vi "PS_set_field_rate.vi"(0 "ramping rate":variant, 1 "set point":variant, 2 "Power supply":T1(ring)) -> ()   [LabVIEW 2020]
panel:
  out "error IO":errorcluster
  in  "error in (no error)":errorcluster
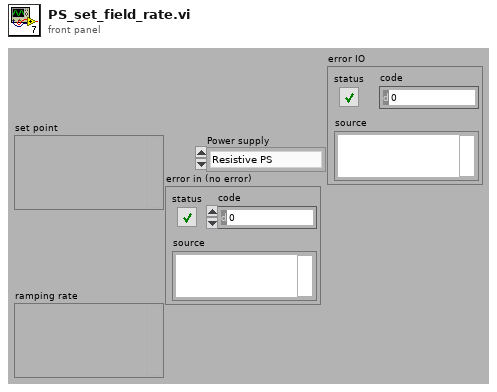
[diagram p1: front panel]
types:
  T1 = enum16{"Resistive PS", "SCM2 PS", "SCM1 PS", "Generic PS", "PPMS"}
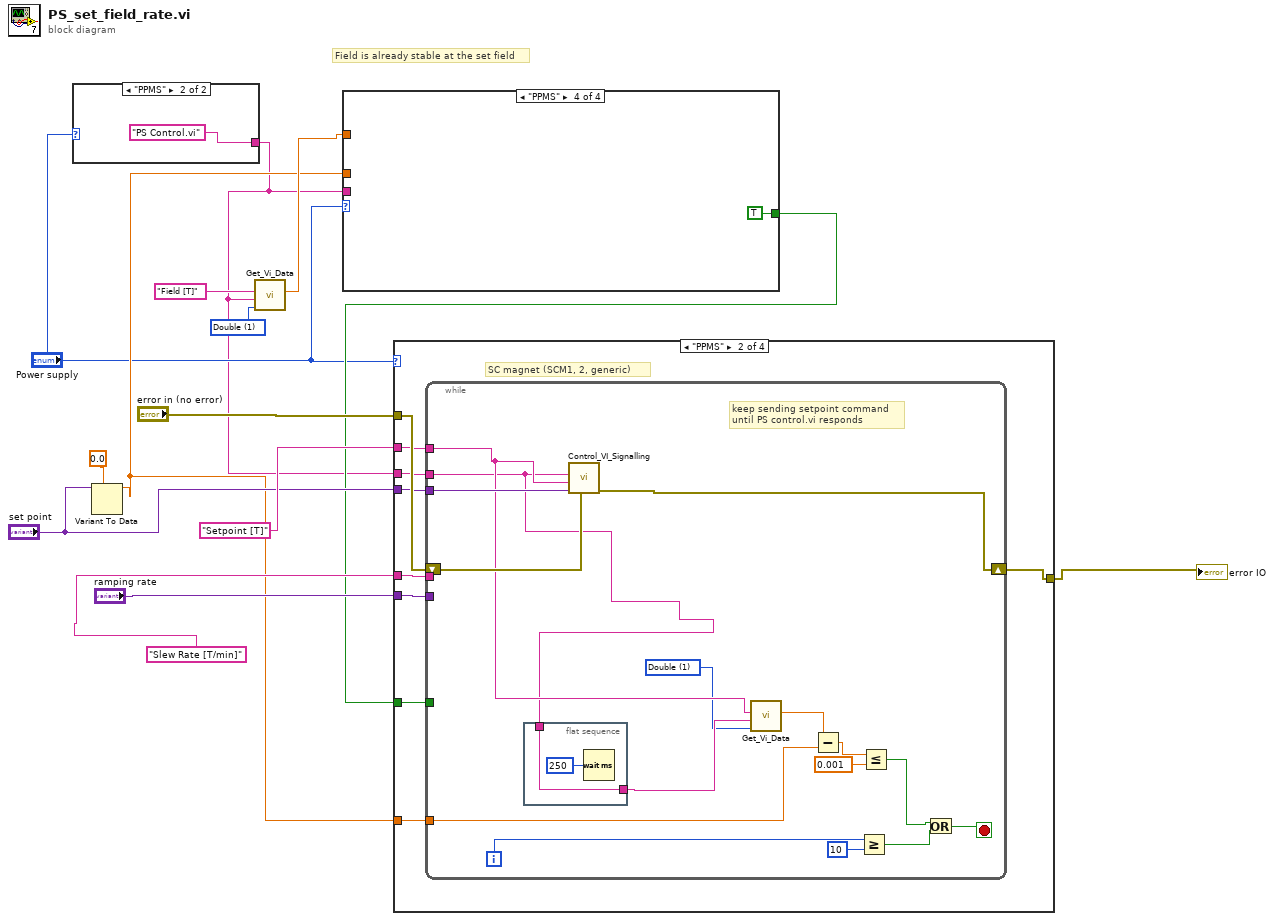
[diagram p0: block diagram]
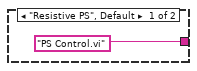
[diagram p2: hidden frame]
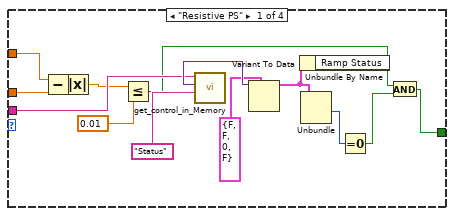
[diagram p3: hidden frame]
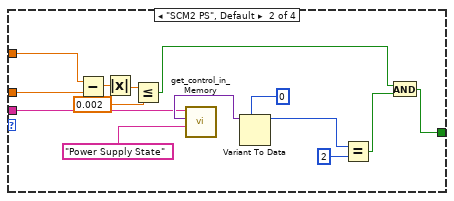
[diagram p4: hidden frame]
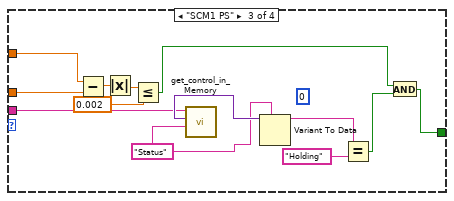
[diagram p5: hidden frame]
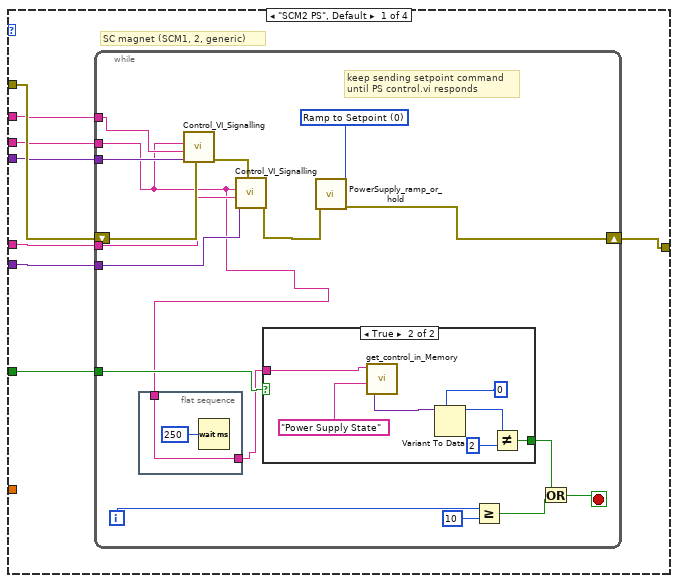
[diagram p6: hidden frame]
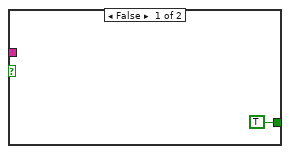
[diagram p7: hidden frame]
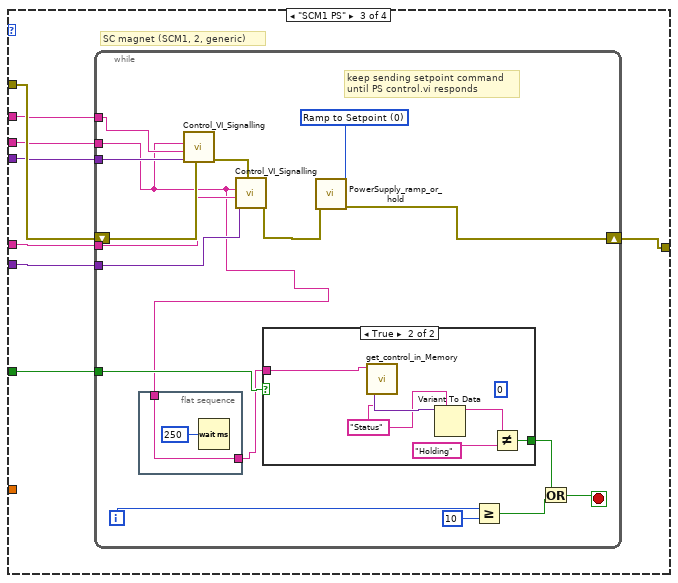
[diagram p8: hidden frame]
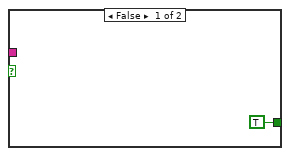
[diagram p9: hidden frame]
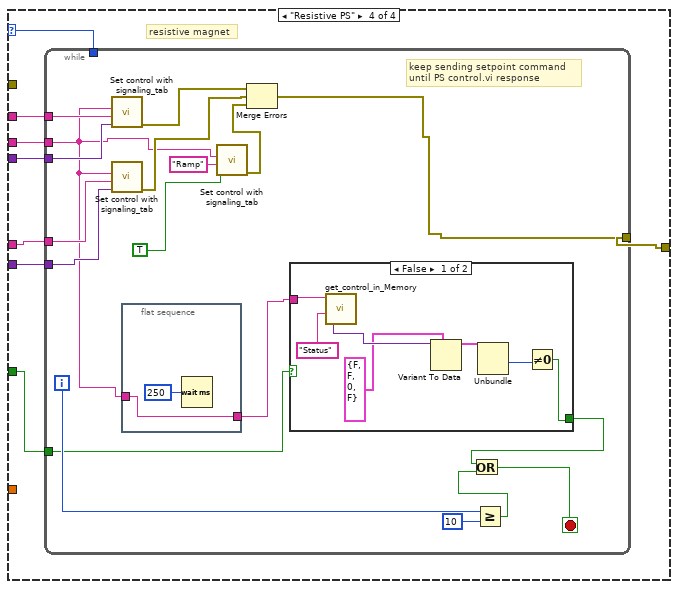
[diagram p10: hidden frame]
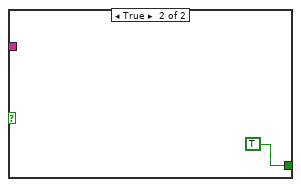
[diagram p11: hidden frame]
diagram:
  w10 = u16 1 items=["String", "Double", "Boolean", "Variant"] ("Data Type")
  # "Field is already stable at the set field"
  n1 = case shown="\"PPMS\"" "Power supply" {
    tunnel: ["PS Control.vi" ("VI name") "PS Control.vi" ("VI name")] -> w1
    frame "Resistive PS", Default {
    }
    frame "PPMS" {
    }
  }
  n2 = Variant To Data(type=0.0, Variant="set point") -> (data=w3:dbl)  [unwired: 1 in, 1 out]
  n3 = call "Get_Vi_Data.vi"("Data Type"=w10, "VI name"=w1, "Control Name"="Field [T]") -> ("Data (Double)"=w6:dbl)  [unwired: 4 in, 4 out]
  n4 = case shown="\"PPMS\"" "Power supply" {
    tunnel: w1 -> [w28 w41 w56 _]
    tunnel: [w27 w37 w54 TRUE] -> w5
    tunnel: w6 -> [w26 w36 w53 _]
    tunnel: w3 -> [w25 w35 w52 _]
    frame "Resistive PS" {
      n5 = Subtract(x=w26, y=w25) -> (x-y=w24:dbl)
      n6 = Absolute Value(x=w24) -> (abs(x)=w20:dbl)
      n7 = Less Or Equal?(x=w20, y=0.01) -> (x <= y?=w22:bool)
      n8 = call "get_control_in_Memory.vi"("Control Name"="Status", "VI Name"=w28) -> ("Value"=w29:variant)  [unwired: 2 in, 1 out]
      n9 = Variant To Data(type=cluster{bool, bool, "Ramp Status":u16, bool} {FALSE, FALSE, "Ramp Status"=0, FALSE} ("Status"), Variant=w29) -> (data=w19:cluster{bool, bool, "Ramp Status":u16, bool})  [unwired: 1 in, 1 out]
      n10 = Unbundle By Name(w19) -> ()  [unwired: 1 out]
      n11 = Unbundle(w19) -> ("Ramp Status"=w18:u16)  [unwired: 3 out]
      n12 = Equal To 0?(x=w18) -> (x = 0?=w17:bool)
      n13 = And(x=w22, y=w17) -> (x .and. y?=w27:bool)
    }
    frame "SCM2 PS", Default {
      n14 = Subtract(x=w36, y=w35) -> (x-y=w34:dbl)
      n15 = Absolute Value(x=w34) -> (abs(x)=w31:dbl)
      n16 = Less Or Equal?(x=w31, y=0.002) -> (x <= y?=w32:bool)
      n17 = call "get_control_in_Memory.vi"("Control Name"="Power Supply State", "VI Name"=w41) -> ("Value"=w43:variant)  [unwired: 2 in, 1 out]
      n18 = Variant To Data(type=0, Variant=w43) -> (data=w39:i32)  [unwired: 1 in, 1 out]
      n19 = Equal?(x=w39, y=2) -> (x = y?=w38:bool)
      n20 = And(x=w32, y=w38) -> (x .and. y?=w37:bool)
    }
    frame "SCM1 PS" {
      (unwired) 0
      w47 = "Status" ("Control Name")
      n21 = Subtract(x=w53, y=w52) -> (x-y=w51:dbl)
      n22 = Absolute Value(x=w51) -> (abs(x)=w48:dbl)
      n23 = Less Or Equal?(x=w48, y=0.002) -> (x <= y?=w49:bool)
      n24 = call "get_control_in_Memory.vi"("Control Name"=w47, "VI Name"=w56) -> ("Value"=w57:variant)  [unwired: 2 in, 1 out]
      n25 = Variant To Data(type=w47, Variant=w57) -> (data=w46:string)  [unwired: 1 in, 1 out]
      n26 = Equal?(x=w46, y="Holding") -> (x = y?=w55:bool)
      n27 = And(x=w49, y=w55) -> (x .and. y?=w54:bool)
    }
    frame "PPMS" {
    }
  }
  n28 = case shown="\"PPMS\"" "Power supply" {
    selector: "Power supply" -> [_ _ _ w159]
    tunnel: "error in (no error)" -> [w66 w102 w128 _]
    tunnel: "Setpoint [T]" ("Control Name") -> [w65 w101 w127 w162]
    tunnel: w1 -> [w64 w100 w126 w161]
    tunnel: "Slew Rate [T/min]" ("Control Name") -> [w63 w99 w125 w160]
    tunnel: "set point" -> [w62 w98 w124 w158]
    tunnel: "ramping rate" -> [w61 w97 w123 w157]
    tunnel: w5 -> [w60 w96 w122 w155]
    tunnel: [w59 w95 w121 w156] -> w4
    tunnel: w3 -> [_ w94 _ _]
    frame "SCM2 PS", Default {
      # "SC magnet (SCM1, 2, generic)"
      n29 = while {
        tunnel: w65 -> [w79]
        tunnel: w64 -> [w73]
        tunnel: w63 -> [w78]
        shift-right: [w80] -> w59
        shift-left: w66 -> [w83]
        tunnel: w62 -> [w77]
        tunnel: w61 -> [w76]
        tunnel: w60 -> [w74]
        i -> [w68]
        stop <- w67 stop-if-true
        w75 = u16 0 items=["Ramp to Setpoint", "Hold"] ("Mode")
        # "keep sending setpoint command\nuntil PS control.vi responds"
        n30 = flat-sequence {
          tunnel: [w84] -> w72
          tunnel: w73 -> [w84]
          frame #0 {
            n31 = Wait (ms)(milliseconds to wait=u32 250) -> ()  [unwired: 1 out]
          }
        }
        n32 = call "Control_VI_Signalling.vi"("error in (no error)"=w83, "Input Value"=w77, "Control Name"=w79, "Target VI name"=w73) -> ("error out"=w82:errorcluster)  [unwired: 7 in]
        n33 = call "Control_VI_Signalling.vi"("error in (no error)"=w82, "Input Value"=w76, "Control Name"=w78, "Target VI name"=w73) -> ("error out"=w81:errorcluster)  [unwired: 7 in]
        n34 = case shown="True" w74 {
          tunnel: [TRUE w88] -> w71
          tunnel: w72 -> [_ w87]
          frame False {
          }
          frame True {
            n35 = call "get_control_in_Memory.vi"("Control Name"="Power Supply State", "VI Name"=w87) -> ("Value"=w92:variant)  [unwired: 2 in, 1 out]
            n36 = Variant To Data(type=0, Variant=w92) -> (data=w90:i32)  [unwired: 1 in, 1 out]
            n37 = Not Equal?(x=w90, y=2) -> (x != y?=w88:bool)
          }
        }
        n38 = call "PowerSupply_ramp_or_hold.vi"("error in (no error)"=w81, "Mode"=w75) -> ("error out"=w80:errorcluster)  [unwired: 9 in]
        n39 = Greater Or Equal?(x=w68, y=10) -> (x >= y?=w69:bool)
        n40 = Or(x=w71, y=w69) -> (x .or. y?=w67:bool)
      }
    }
    frame "PPMS" {
      # "SC magnet (SCM1, 2, generic)"
      n41 = while {
        tunnel: w101 -> [w111]
        tunnel: w100 -> [w103]
        tunnel: w99 -> [_]
        shift-right: [w115] -> w95
        shift-left: w102 -> [w118]
        tunnel: w98 -> [w117]
        tunnel: w97 -> [_]
        tunnel: w96 -> [_]
        tunnel: w94 -> [w108]
        i -> [w116]
        stop <- w104 stop-if-true
        w110 = u16 1 items=["String", "Double", "Boolean", "Variant"] ("Data Type")
        # "keep sending setpoint command\nuntil PS control.vi responds"
        n42 = flat-sequence {
          tunnel: [w119] -> w112
          tunnel: w103 -> [w119]
          frame #0 {
            n43 = Wait (ms)(milliseconds to wait=u32 250) -> ()  [unwired: 1 out]
          }
        }
        n44 = call "Control_VI_Signalling.vi"("error in (no error)"=w118, "Input Value"=w117, "Control Name"=w111, "Target VI name"=w103) -> ("error out"=w115:errorcluster)  [unwired: 7 in]
        n45 = call "Get_Vi_Data.vi"("Data Type"=w110, "VI name"=w112, "Control Name"=w111) -> ("Data (Double)"=w109:dbl)  [unwired: 4 in, 4 out]
        n46 = Subtract(x=w109, y=w108) -> (x-y=w107:dbl)
        n47 = Greater Or Equal?(x=w116, y=10) -> (x >= y?=w113:bool)
        n48 = Less Or Equal?(x=w107, y=0.001) -> (x <= y?=w105:bool)
        n49 = Or(x=w105, y=w113) -> (x .or. y?=w104:bool)
      }
    }
    frame "SCM1 PS" {
      # "SC magnet (SCM1, 2, generic)"
      n50 = while {
        tunnel: w127 -> [w141]
        tunnel: w126 -> [w135]
        tunnel: w125 -> [w140]
        shift-right: [w142] -> w121
        shift-left: w128 -> [w145]
        tunnel: w124 -> [w139]
        tunnel: w123 -> [w138]
        tunnel: w122 -> [w136]
        i -> [w130]
        stop <- w129 stop-if-true
        w137 = u16 0 items=["Ramp to Setpoint", "Hold"] ("Mode")
        # "keep sending setpoint command\nuntil PS control.vi responds"
        n51 = flat-sequence {
          tunnel: [w146] -> w134
          tunnel: w135 -> [w146]
          frame #0 {
            n52 = Wait (ms)(milliseconds to wait=u32 250) -> ()  [unwired: 1 out]
          }
        }
        n53 = call "Control_VI_Signalling.vi"("error in (no error)"=w145, "Input Value"=w139, "Control Name"=w141, "Target VI name"=w135) -> ("error out"=w144:errorcluster)  [unwired: 7 in]
        n54 = call "Control_VI_Signalling.vi"("error in (no error)"=w144, "Input Value"=w138, "Control Name"=w140, "Target VI name"=w135) -> ("error out"=w143:errorcluster)  [unwired: 7 in]
        n55 = case shown="True" w136 {
          tunnel: [TRUE w152] -> w133
          tunnel: w134 -> [_ w151]
          frame False {
          }
          frame True {
            (unwired) 0
            w150 = "Status" ("Control Name")
            n56 = call "get_control_in_Memory.vi"("Control Name"=w150, "VI Name"=w151) -> ("Value"=w154:variant)  [unwired: 2 in, 1 out]
            n57 = Variant To Data(type=w150, Variant=w154) -> (data=w153:string)  [unwired: 1 in, 1 out]
            n58 = Not Equal?(x=w153, y="Holding" ("Control Name")) -> (x != y?=w152:bool)
          }
        }
        n59 = call "PowerSupply_ramp_or_hold.vi"("error in (no error)"=w143, "Mode"=w137) -> ("error out"=w142:errorcluster)  [unwired: 9 in]
        n60 = Greater Or Equal?(x=w130, y=10) -> (x >= y?=w131:bool)
        n61 = Or(x=w133, y=w131) -> (x .or. y?=w129:bool)
      }
    }
    frame "Resistive PS" {
      # "resistive magnet"
      n62 = while {
        tunnel: [w169] -> w156
        tunnel: w162 -> [w175]
        tunnel: w161 -> [w166]
        tunnel: w160 -> [w174]
        tunnel: w159 -> [_]
        tunnel: w158 -> [w168]
        tunnel: w157 -> [w167]
        tunnel: w155 -> [w164]
        i -> [w173]
        stop <- w170 stop-if-true
        # "keep sending setpoint command\nuntil PS control.vi response"
        n63 = call "Set control with signaling_tab.vi"("Value (Signaling)"=w168, "Control Name"=w175, "VI Name"=w166) -> ("error out"=w178:errorcluster)  [unwired: 8 in]
        n64 = call "Set control with signaling_tab.vi"("Value (Signaling)"=w167, "Control Name"=w174, "VI Name"=w166) -> ("error out"=w177:errorcluster)  [unwired: 8 in]
        n65 = flat-sequence {
          tunnel: [w181] -> w165
          tunnel: w166 -> [w181]
          frame #0 {
            n66 = Wait (ms)(milliseconds to wait=u32 250) -> ()  [unwired: 1 out]
          }
        }
        n67 = call "Set control with signaling_tab.vi"("Value (Signaling)"=TRUE, "Control Name"="Ramp", "VI Name"=w166) -> ("error out"=w176:errorcluster)  [unwired: 8 in]
        n68 = Merge Errors(w178, w177, w176) -> (w169:errorcluster)
        n69 = case shown="False" w164 {
          tunnel: w165 -> [w184 _]
          tunnel: [w183 TRUE] -> w163
          frame False {
            n70 = call "get_control_in_Memory.vi"("Control Name"="Status", "VI Name"=w184) -> ("Value"=w188:variant)  [unwired: 2 in, 1 out]
            n71 = Variant To Data(type=cluster{bool, bool, "Ramp Status":u16, bool} {FALSE, FALSE, "Ramp Status"=0, FALSE} ("Status"), Variant=w188) -> (data=w189:cluster{bool, bool, "Ramp Status":u16, bool})  [unwired: 1 in, 1 out]
            n72 = Unbundle(w189) -> ("Ramp Status"=w185:u16)  [unwired: 3 out]
            n73 = Not Equal To 0?(x=w185) -> (x != 0?=w183:bool)
          }
          frame True {
          }
        }
        n74 = Greater Or Equal?(x=w173, y=10) -> (x >= y?=w171:bool)
        n75 = Or(x=w163, y=w171) -> (x .or. y?=w170:bool)
      }
    }
  }
  "error IO" <- w4
